vi "Encoder_RefNum Registry Close.vi"(1 "error in (no error)":errorcluster, 2 "RobotEncoderRef":T5) -> (0 "error out":errorcluster)   [LabVIEW 2013]
uses:
  <vilib>/Rock Robotics/WPI/Encoder/WPI_EncoderDevRef.ctl
  <vilib>/Rock Robotics/SystemInterfaces/Encoder/FPGA_EncoderIdx.ctl
  <vilib>/Rock Robotics/SystemInterfaces/Counter/FPGA_CounterCtrSystemIndex.ctl
  <vilib>/Rock Robotics/WPI/Encoder/WPI_EncoderType.ctl
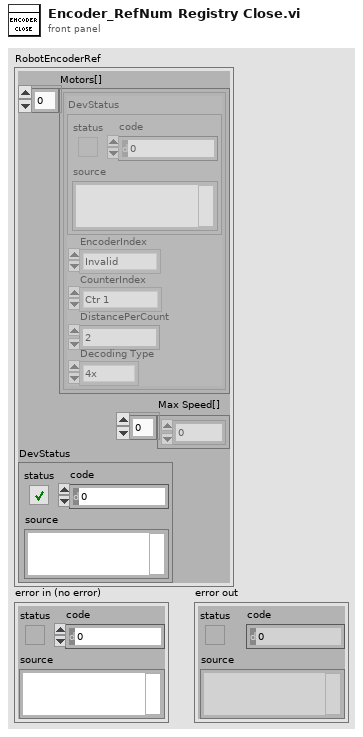
[diagram p1: front panel]
types:
  T1 = typedef "WPI_EncoderDevRef.ctl" = cluster{"DevStatus":errorcluster, "EncoderIndex":T2, "CounterIndex":T3, "DistancePerCount":dbl, "Decoding Type":T4}
  T2 = typedef "FPGA_EncoderIdx.ctl" = enum8{"Enc 0", "Enc 1", "Enc 2", "Enc 3", "Invalid"}
  T3 = typedef "FPGA_CounterCtrSystemIndex.ctl" = enum8{"Ctr 0", "Ctr 1", "Ctr 2", "Ctr 3", "Ctr 4", "Ctr 5", "Ctr 6", "Ctr 7", "Invalid"}
  T4 = typedef "WPI_EncoderType.ctl" = enum16{"1x", "2x", "4x"}
  T5 = cluster{"Motors[]":T1[], "DevStatus":errorcluster, "Max Speed[]":dbl[]}
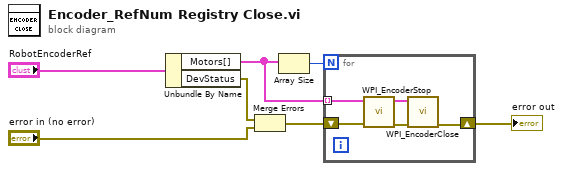
[diagram p0: block diagram]
diagram:
  n1 = Unbundle By Name("RobotEncoderRef") -> ("Motors[]"=w5:T1[], "DevStatus"=w4:errorcluster)
  n2 = Merge Errors(w4, "error in (no error)") -> (w2:errorcluster)
  n3 = Array Size(array=w5) -> (size(s)=w6:i32)
  n4 = for {
    N: w6 -> [_]
    tunnel: w5 -> [w10] mode=indexing
    shift-right: [w8] -> w1
    shift-left: w2 -> [w9]
    n5 = call <vilib>:"WPI_EncoderStop.vi"("error in (no error)"=w9, "EncoderDevRef"=w10) -> ("error out"=w12:errorcluster, "EncoderDevRef"=w11:T1)  [unwired: 8 in]
    n6 = call <vilib>:"WPI_EncoderClose.vi"("error in (no error)"=w12, "EncoderDevRef"=w11) -> ("error out"=w8:errorcluster)  [unwired: 9 in]
  }
  "error out" <- w1
